vi "CtrlSignalValue.vi"(1 "error in":errorcluster, 2 "data string":string, 3 "variant":variant, 4 "reference":refnum<vi>) -> (0 "error out":errorcluster)   [LabVIEW 2014]
doc: "Sets the value of a front-panel control.\nParameters:\nany:ctrl, Ctrl.\nany:value, new value for control/indicator.\nErrors:\nNot a Ctrl.\nData type of value does not match data type of control/indicator.\nData type of control/indicator not supported."
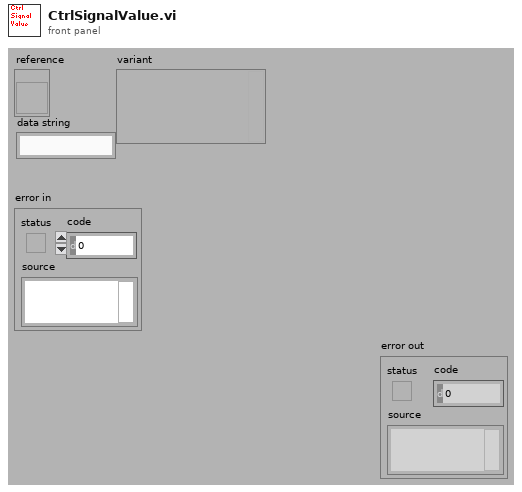
[diagram p1: front panel]
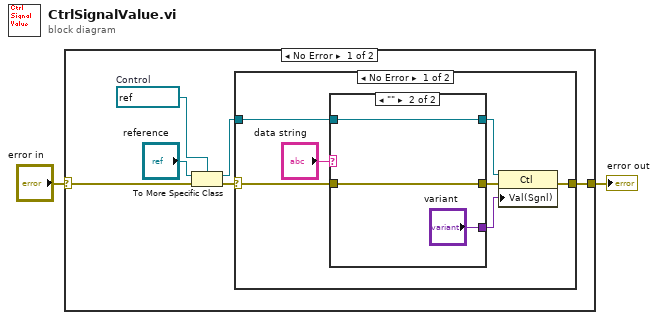
[diagram p0: block diagram]
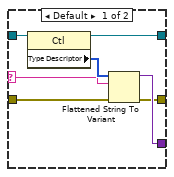
[diagram p2: hidden frame]
diagram:
  n1 = case shown="No Error" "error in" {
    selector: "error in" -> [w4 w27]
    tunnel: [w8 w27] -> w2
    frame No Error {
      w6 = refnum<vi> refnum  # Control
      n2 = To More Specific Class(target class=w6, reference="reference", error in=w4) -> (specific class reference=w5:refnum<vi>, error out=w3:errorcluster)
      n3 = case shown="No Error" w3 {
        selector: w3 -> [w10 w26]
        tunnel: [w15 w26] -> w8
        tunnel: w5 -> [w13 _]
        frame No Error {
          n4 = case shown="\"\"" "data string" {
            selector: "data string" -> [w20 _]
            tunnel: w13 -> [w22 w25]
            tunnel: [w19 "variant"] -> w12
            tunnel: [w18 w25] -> w11
            tunnel: w10 -> [w17 w23]
            tunnel: [w16 w23] -> w9
            frame Default {
              n5 = property class="Ctl"(reference=w22) -> (reference out=w18:refnum<vi>, "Type Descriptor"=w21:i16[])  [unwired: 1 in, 1 out]
              n6 = Flattened String To Variant(4:w17, 6:w20, 7:w21) -> (0:w16:errorcluster, 3:w19:variant)
            }
            frame "" {
            }
          }
          n7 = property class="Ctl"(reference=w11, error in=w9, "Val(Sgnl)"=w12) -> (error out=w15:errorcluster)  [unwired: 1 out]
        }
        frame Error {
        }
      }
    }
    frame Error {
    }
  }
  "error out" <- w2
